vi "updateResultsBox.vi"(8 "error in (no error)":errorcluster, 10 "results":T1, 11 "AnalysisResultsViewer in":refnum<class "AnalysisResultsViewer.lvclass">) -> (0 "error out":errorcluster, 3 "AnalysisResultsViewer out":refnum<class "AnalysisResultsViewer.lvclass">)   [LabVIEW 2011, in "Views.lvlib" / "Camera.lvlib" / "AnalysisResultsViewer.lvclass"]
uses:
  AnalysisResultsViewer.lvclass
  AnalysisResultsViewer.lvclass/AnalysisResultsViewer.ctl
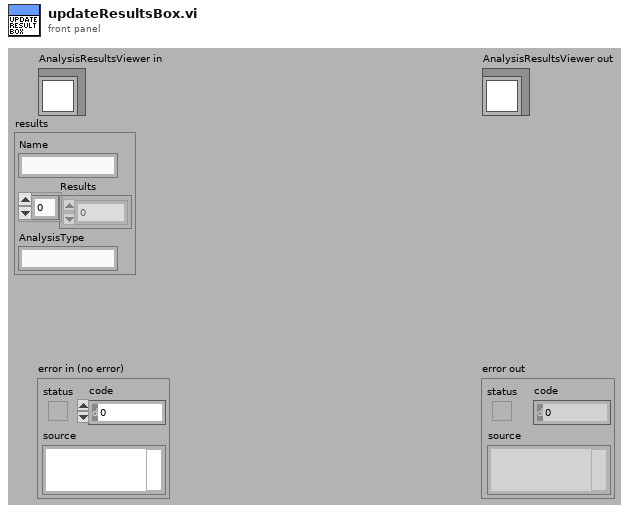
[diagram p1: front panel]
types:
  T1 = cluster{"Name":string, "Results":dbl[], "AnalysisType":string}
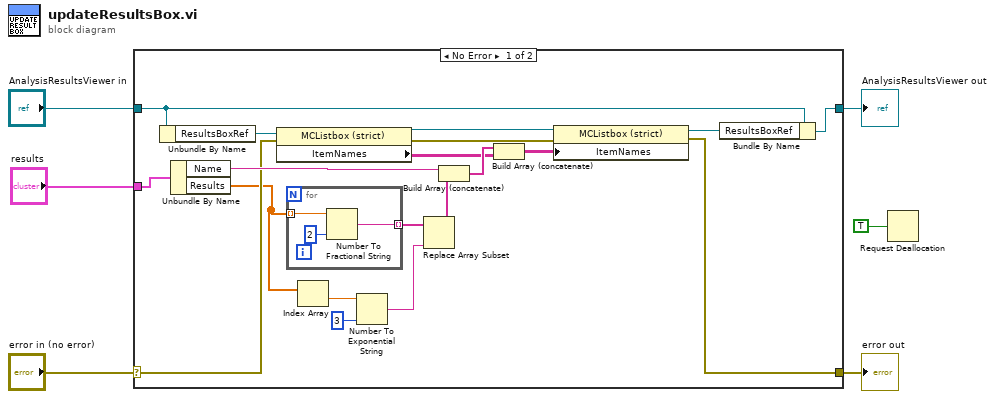
[diagram p0: block diagram]
diagram:
  n1 = case shown="No Error" "error in (no error)" {
    selector: "error in (no error)" -> [w15 w30]
    tunnel: [w16 w30] -> w5
    tunnel: [w13 w29] -> w3
    tunnel: "AnalysisResultsViewer in" -> [w14 w29]
    tunnel: "results" -> [w25 _]
    frame No Error {
      n2 = Unbundle By Name(w14) -> ("ResultsBoxRef"=w24:refnum<vi>)
      n3 = Unbundle By Name(w25) -> ("Name"=w23:string, "Results"=w12:dbl[])
      n4 = property class="MCListbox (strict)"(reference=w24, error in=w15) -> (reference out=w20:refnum<vi>, error out=w19:errorcluster, "ItemNames"=w21:string[][])
      n5 = for {
        tunnel: w12 -> [w28] mode=indexing
        tunnel: [w27] -> w9 mode=indexing
        n6 = Number To Fractional String(number=w28, precision (6)=2) -> (F-format string=w27:string)  [unwired: 2 in]
      }
      n7 = Index Array(array=w12) -> (element=w11:dbl)  [unwired: 1 in]
      n8 = Number To Exponential String(number=w11, precision (6)=3) -> (E-format string=w8:string)  [unwired: 2 in]
      n9 = Replace Array Subset(array=w9, new element=w8) -> (w7:string[])  [unwired: 1 in]
      n10 = Build Array (concatenate)(w23, w7) -> (w22:string[])
      n11 = Build Array (concatenate)(w22, w21) -> (w18:string[][])
      n12 = property class="MCListbox (strict)"(reference=w20, error in=w19, "ItemNames"=w18) -> (reference out=w17:refnum<vi>, error out=w16:errorcluster)
      n13 = Bundle By Name(cluster=w14, "ResultsBoxRef"=w17) -> (w13:refnum<class "AnalysisResultsViewer.lvclass">)
    }
    frame Error {
    }
  }
  "error out" <- w5
  "AnalysisResultsViewer out" <- w3
  n14 = Request Deallocation(TRUE ("flag")) -> ()
